vi "SV Read Next Overlapping Data.vi"(5 "overlap (50 %)":dbl=50.0 min=0.0 max=100.0 step=1.0, 6 "reset start (F)":bool, 7 "reader ID":string="OverlappingData", 8 "error in (no error)":errorcluster, 9 "timeout (0 ms)":i32, 10 "block length (4096 samples)":i32=4096, 11 "buffer":refnum<data-value>) -> (0 "error out":errorcluster, 1 "end of buffer":bool, 2 "waveforms subset":waveform(dbl)[](array[waveform]), 3 "buffer out":refnum<data-value>)   [LabVIEW 2017]
doc: "Adds buffering to stimulus-response applications. You must manually select the polymorphic instance to use."
uses:
  <vilib>/addons/_NISVFA/_Shared subVIs/Data Objects/Waveforms (DBL)/Waveforms (N Ch).lvclass
  C:/Program Files (x86)/National Instruments/LabVIEW 2017/vi.lib/addons/_NISVFA/_Shared subVIs/Data Objects/Data/Data.lvclass
  <vilib>/addons/_NISVFA/_Shared subVIs/Data Objects/Data/Data.lvclass/Data.ctl
  <vilib>/addons/_NISVFA/_Shared subVIs/Data Objects/Waveforms (DBL)/Waveforms (N Ch).lvclass/Waveforms (N Ch).ctl
  <vilib>/addons/_NISVFA/_Shared subVIs/Data Objects/Waveforms (DBL)/Read Mode for Deleting Stale Data.vi
  <vilib>/addons/_NISVFA/_Shared subVIs/Data Objects/subVIs/Get Data Timestamp.vi
  <vilib>/addons/_NISVFA/_Shared subVIs/Common/sv_Convert Timestamp to Relative Index.vi
  <vilib>/addons/_NISVFA/_Shared subVIs/Data Objects/subVIs/Get Data Length.vi
  <vilib>/addons/_NISVFA/_Shared subVIs/Common/SV Get Data Subset.vi
  <vilib>/addons/_NISVFA/_Shared subVIs/Common/svc_Copy Waveform Subset (Index).vi
  <vilib>/addons/_NISVFA/_Shared subVIs/Common/sv_Get NI Property Name String.vi
  <vilib>/addons/_NISVFA/_Shared subVIs/Data Objects/subVIs/Get Oldest of ReaderTimestamps.vi
  <vilib>/addons/_NISVFA/_Shared subVIs/Data Objects/subVIs/Set Data Timestamp.vi
  <vilib>/addons/_NISVFA/_Shared subVIs/Data Objects/subVIs/Set Data Length.vi
  <vilib>/addons/_NISVFA/_Shared subVIs/Common/svc_Get Waveform Subset (Index).vi
  <vilib>/addons/_NISVFA/_Shared subVIs/Common/svc_Copy Array Subset (Index).vi
  <vilib>/addons/_NISVFA/_Shared subVIs/Common/svc_Get Array Subset (Index).vi
  <vilib>/addons/_NISVFA/_Shared subVIs/Common/svc_Coerce Index and Length.vi
  <vilib>/addons/_NISVFA/_Shared subVIs/Common/svc_Conditional Merge Error.vi
  <vilib>/Utility/error.llb/Trim Whitespace.vi
  <vilib>/addons/_NISVFA/_Shared subVIs/Data Objects/Data/Data.lvclass
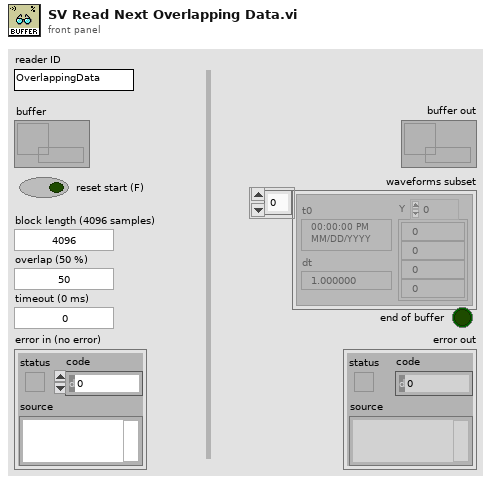
[diagram p1: front panel]
types:
  T1 = enum16{"Data Ready", "First Sample Not Yet Available", "Last Sample Not Yet Available", "Data No Longer Available"}
  T2 = typedef "svc_Delete Data Options (enum).ctl" = enum16{"Write", "Read", "Release"}
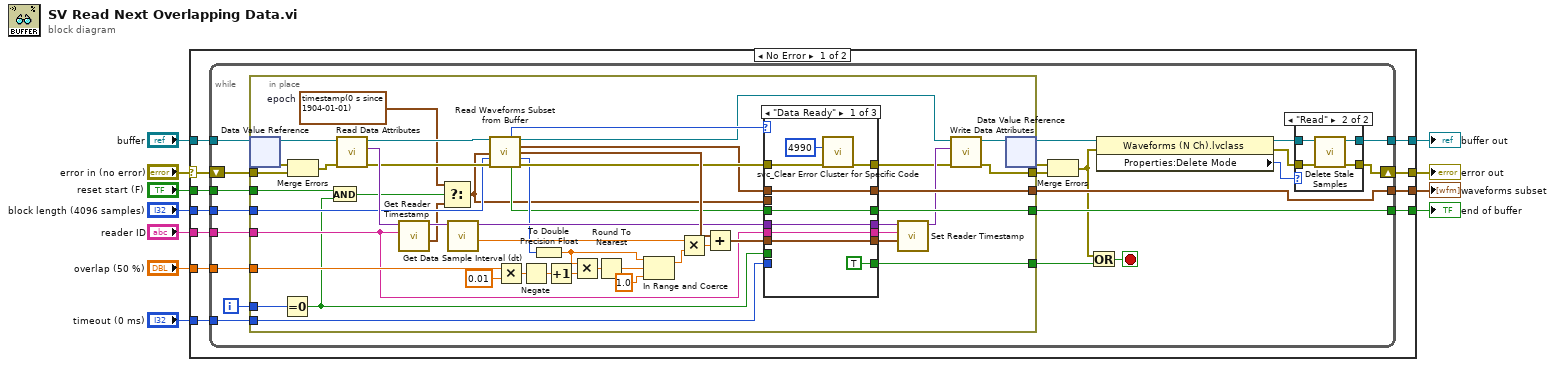
[diagram p0: block diagram]
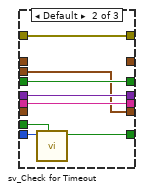
[diagram p3: hidden frame]
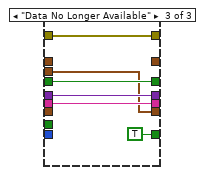
[diagram p4: hidden frame]
diagram:
  n1 = case shown="No Error" "error in (no error)" {
    selector: "error in (no error)" -> [w16 w122]
    tunnel: "overlap (50 %)" -> [w22 _]
    tunnel: "buffer" -> [w15 w123]
    tunnel: "reset start (F)" -> [w21 _]
    tunnel: [w14 w123] -> w8
    tunnel: "block length (4096 samples)" -> [w20 _]
    tunnel: [w13 w122] -> w6
    tunnel: [w19 _] -> w5
    tunnel: [w18 _] -> w4
    tunnel: "reader ID" -> [w17 _]
    tunnel: "timeout (0 ms)" -> [w12 _]
    frame No Error {
      n2 = while {
        tunnel: w22 -> [w43]
        tunnel: w21 -> [w42]
        tunnel: w20 -> [w41]
        tunnel: [w26] -> w19
        tunnel: [w40] -> w18
        tunnel: w17 -> [w39]
        tunnel: w15 -> [w37]
        tunnel: [w27] -> w14
        shift-right: [w28] -> w13
        shift-left: w16 -> [w38]
        tunnel: w12 -> [w34]
        i -> [w33]
        stop <- w24 stop-if-true
        n3 = in-place {
          in-place-border: w43 -> [w98]
          in-place-border: w42 -> [w52]
          in-place-border: w41 -> [w83]
          in-place-border: [w59] -> w35
          in-place-border: [w73] -> w26
          in-place-border: [w72] -> w40
          in-place-border: w39 -> [w69]
          in-place-border: w38 -> [w66]
          in-place-border: w34 -> [w64]
          in-place-border: w33 -> [w53]
          in-place-border: [w63] -> w23
          w88 = timestamp(0 s since 1904-01-01)  # epoch
          n4 = in-place-dvr #1(w37) -> (w68:refnum<class "Waveforms (N Ch).lvclass">, w67:errorcluster)
          n5 = Equal To 0?(x=w53) -> (x = 0?=w51:bool)
          n6 = Merge Errors(w67, w66) -> (w65:errorcluster)
          n7 = And(x=w52, y=w51) -> (x .and. y?=w50:bool)
          n8 = call <vilib>:"Read Data Attributes.vi"("error in (no error)"=w65, "Data in"=w68) -> ("error out"=w89:errorcluster, "data attributes"=w91:variant, "Data out"=w90:refnum<class "Waveforms (N Ch).lvclass">)  [unwired: 7 in]
          n9 = call <vilib>:"Get Reader Timestamp.vi"("ID"=w69, "data attributes"=w91) -> ("timestamp"=w70:timestamp, "data attributes"=w86:variant)  [unwired: 8 in]
          n10 = Select(t=w88, s=w50, f=w70) -> (s? t:f=w54:timestamp)
          n11 = call <vilib>:"Get Data Sample Interval (dt).vi"("variant in"=w86) -> ("dt [s]"=w84:dbl, "variant out"=w85:variant)  [unwired: 9 in]
          n12 = call <vilib>:"Read Waveforms Subset from Buffer.vi"("Waveforms (N Ch)"=w90, "timestamp"=w54, "block length"=w83, "error in (no error)"=w89) -> ("subset status"=w75:T1, "Waveforms (N Ch)"=w61:refnum<class "Waveforms (N Ch).lvclass">, "waveforms subset"=w74:waveform(dbl)[], "actual timestamp"=w87:timestamp, "actual length"=w76:i32, "end of buffer"=w71:bool, "error out"=w77:errorcluster)  [unwired: 5 in]
          n13 = Multiply(x=w98, y=0.01) -> (x*y=w96:dbl)
          n14 = Negate(x=w96) -> (-x=w95:dbl)
          n15 = To Double Precision Float(number=w76) -> (double precision float=w82:dbl)
          n16 = Increment(x=w95) -> (x+1=w92:dbl)
          n17 = Multiply(x=w82, y=w92) -> (x*y=w94:dbl)
          n18 = Round To Nearest(number=w94) -> (nearest integer value=w81:dbl)
          n19 = In Range and Coerce(upper limit=w82, x=w81, lower limit=1.0) -> (coerced(x)=w80:dbl)  [unwired: 1 out]
          n20 = Multiply(x=w84, y=w80) -> (x*y=w79:dbl)
          n21 = Add(x=w87, y=w79) -> (x+y=w78:timestamp)
          n22 = case shown="\"Data Ready\"" w75 {
            tunnel: w69 -> [w99 w110 w117]
            tunnel: w85 -> [w101 w111 w118]
            tunnel: w78 -> [w100 _ _]
            tunnel: w77 -> [w104 w115 w121]
            tunnel: [w103 w115 w121] -> w58
            tunnel: w74 -> [w107 _ _]
            tunnel: [w107 _ _] -> w73
            tunnel: w71 -> [w106 w114 w120]
            tunnel: [w106 w114 w120] -> w72
            tunnel: w64 -> [_ w113 _]
            tunnel: [TRUE ("timeout") w112 TRUE ("timeout")] -> w63
            tunnel: [w101 w111 w118] -> w57
            tunnel: [w100 w109 w116] -> w56
            tunnel: [w99 w110 w117] -> w55
            tunnel: w54 -> [_ w109 w116]
            tunnel: w51 -> [_ w108 _]
            frame "Data Ready" {
              n23 = call <vilib>:"svc_Clear Error Cluster for Specific Code.vi"("error in (no error)"=w104, "code"=4990) -> ("error out"=w103:errorcluster)  [unwired: 12 in, 1 out]
            }
            frame Default {
              n24 = call <vilib>:"sv_Check for Timeout.vi"("reset"=w108, "timeout [ms]"=w113) -> ("timeout"=w112:bool)  [unwired: 8 in, 1 out]
            }
            frame "Data No Longer Available" {
            }
          }
          n25 = call <vilib>:"Set Reader Timestamp.vi"("timestamp"=w56, "ID"=w55, "data attributes in"=w57) -> ("data attributes out"=w62:variant)  [unwired: 8 in]
          n26 = call <vilib>:"Write Data Attributes.vi"("error in (no error)"=w58, "data attributes"=w62, "Data in"=w61) -> ("error out"=w59:errorcluster, "Data out"=w60:refnum<class "Waveforms (N Ch).lvclass">)  [unwired: 7 in]
          n27 = in-place-dvr #1(w60) -> (w29:refnum<data-value>, w36:errorcluster)
        }
        n28 = Merge Errors(w36, w35) -> (w25:errorcluster)
        n29 = Or(x=w25, y=w23) -> (x .or. y?=w24:bool)
        n30 = property class="Waveforms (N Ch).lvclass"(reference=w29, error in=w25) -> (reference out=w31:refnum<data-value>, error out=w30:errorcluster, "Properties:Delete Mode"=w32:T2)
        n31 = case shown="\"Read\"" w32 {
          tunnel: [w45 w48] -> w27
          tunnel: w31 -> [w45 w49]
          tunnel: w30 -> [w44 w47]
          tunnel: [w44 w46] -> w28
          frame Default {
          }
          frame "Read" {
            n32 = call <vilib>:"Delete Stale Samples.vi"("error in (no error)"=w47, "buffer"=w49) -> ("error out"=w46:errorcluster, "buffer"=w48:refnum<data-value>)  [unwired: 6 in, 2 out]
          }
        }
      }
    }
    frame Error {
    }
  }
  "error out" <- w6
  "waveforms subset" <- w5
  "buffer out" <- w8
  "end of buffer" <- w4
